vi "open new fpga reference.vi"(8 "error in":errorcluster, 11 "io configuration in":refnum<class "io configuration.lvclass">) -> (0 "error out":errorcluster, 1 "Load FPGA":bool, 2 "Bitfile reference out":refnum<k20>, 3 "io configuration out":refnum<class "io configuration.lvclass">)   [LabVIEW 2014, in "io configuration.lvclass"]
doc: "Opens a new VI reference based on the configured system. Calling code is responsible for closing this reference."
uses:
  io configuration.lvclass
  <vilib>/NI/Tag Bus Module Framework/FPGA manager/FPGA manager.lvlib
  <vilib>/NI/Tag Bus Module Framework/FPGA manager/methods.ctl
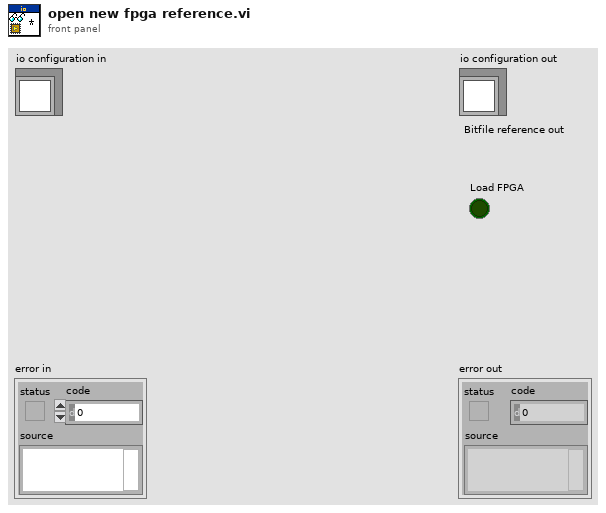
[diagram p1: front panel]
types:
  T1 = typedef "FPGA manager.lvlib/methods.ctl" = enum16{"initialize bitfile", "cache bitfile", "locate bitfile", "close bitfile", "clear manager"}
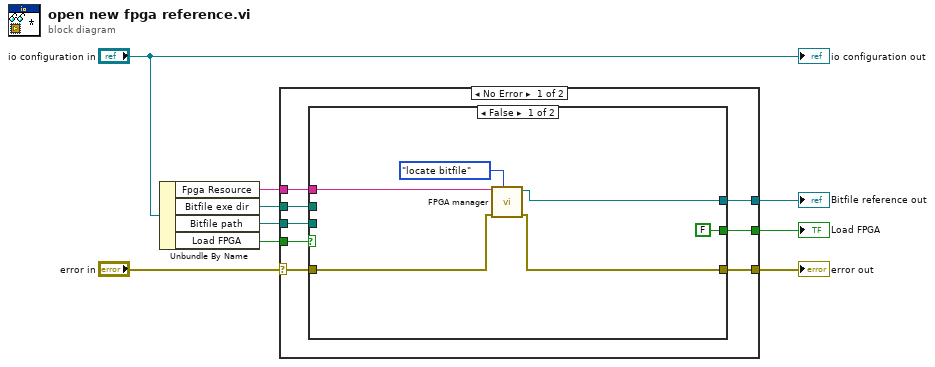
[diagram p0: block diagram]
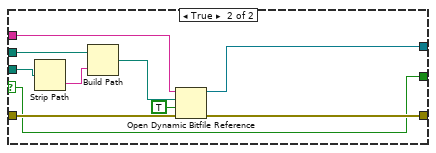
[diagram p2: hidden frame]
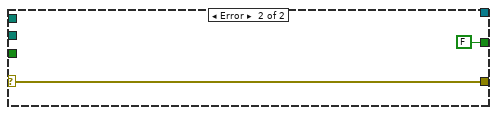
[diagram p3: hidden frame]
diagram:
  n1 = Unbundle By Name("io configuration in") -> ("Fpga Resource"=w5:string, "Bitfile exe dir"=w6:path, "Bitfile path"=w3:path, "Load FPGA"=w2:bool)
  n2 = case shown="No Error" "error in" {
    selector: "error in" -> [w17 w35]
    tunnel: w6 -> [w14 _]
    tunnel: [w16 w35] -> w7
    tunnel: w5 -> [w13 _]
    tunnel: [w15 _] -> w4
    tunnel: w2 -> [w12 _]
    tunnel: w3 -> [w11 _]
    tunnel: [w10 FALSE] -> w1
    frame No Error {
      n3 = case shown="False" w12 {
        selector: w12 -> [_ w24]
        tunnel: w17 -> [w22 w33]
        tunnel: [w21 w32] -> w16
        tunnel: [w19 w31] -> w15
        tunnel: w14 -> [_ w28]
        tunnel: w13 -> [w20 w30]
        tunnel: w11 -> [_ w27]
        tunnel: [FALSE w24] -> w10
        frame False {
          n4 = call <vilib>:"FPGA manager.vi"("action"=methods."locate bitfile", "error in"=w22, "RIO resource"=w20) -> ("error out"=w21:errorcluster, "bitfile"=w19:refnum<k20>)  [unwired: 6 in, 1 out]
        }
        frame True {
          n5 = Strip Path(path=w27) -> (name=w26:string)  [unwired: 1 out]
          n6 = Build Path(base path=w28, name or relative path=w26) -> (appended path=w25:path)
          n7 = Open Dynamic Bitfile Reference(0:w30, 1:w25, 2:TRUE ("Run When Loaded"), 3:w33) -> (5:w31:refnum<k20>, 8:w32:errorcluster)  [unwired: 1 in]
        }
      }
    }
    frame Error {
    }
  }
  "error out" <- w7
  "Bitfile reference out" <- w4
  "Load FPGA" <- w1
  "io configuration out" <- "io configuration in"
